vi "3D-SaveVersionParams.vi"(9 "Pic Param  Data Collect":string[][](table)=[["", "", ""], ["", "", ""]], 10 "名称或相对路径":string, 11 "路径":path) -> ()   [LabVIEW 2017]
uses:
  <vilib>/Utility/file.llb/Write To Spreadsheet File (string).vi
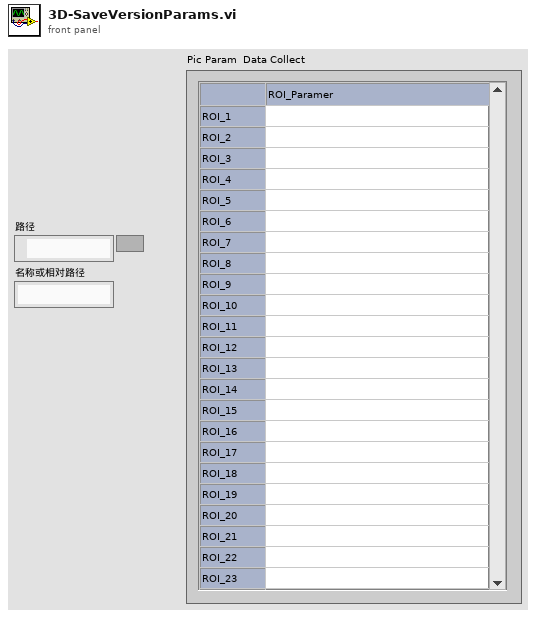
[diagram p1: front panel]
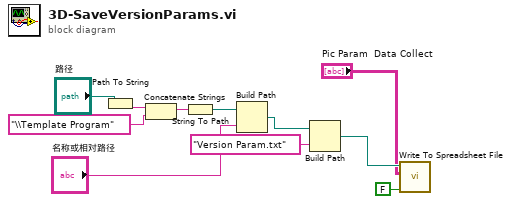
[diagram p0: block diagram]
diagram:
  n1 = Path To String(path="路径") -> (string=w11:string)
  n2 = Concatenate Strings(w11, "\\Template Program" ("字符串")) -> (w10:string)
  n3 = String To Path(string=w10) -> (path=w8:path)
  n4 = Build Path(base path=w8, name or relative path="名称或相对路径") -> (appended path=w5:path)
  n5 = Build Path(base path=w5, name or relative path="Version Param.txt" ("名称或相对路径")) -> (appended path=w2:path)
  n6 = call-poly <vilib>:"Write To Spreadsheet File.vi"("append to file? (new file:F)"=FALSE, "2D data"="Pic Param  Data Collect", "file path (dialog if empty)"=w2) -> ()  [unwired: 5 in, 1 out]
